vi "New Server Thread.vi"(1 "connection ID":refnum<k5>) -> (0 "Server Thread":cluster{"connection ID":refnum<k5>})   [LabVIEW 2016]
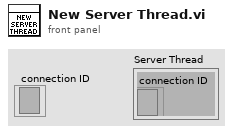
[diagram p1: front panel]
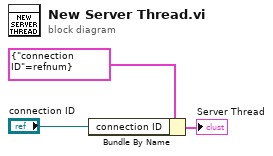
[diagram p0: block diagram]
diagram:
  n1 = Bundle By Name(cluster=cluster{"connection ID":refnum<k5>} {"connection ID"=refnum}, "connection ID"="connection ID") -> (→"Server Thread":cluster{"connection ID":refnum<k5>})
